vi "testarrayofclusters.vi"() -> ()   [LabVIEW 2011]
uses:
  LV JSON.lvlib
panel:
  out "Array of clusters out":T1(array[cluster])
  out "Array of clusters OK?":bool
  out "Array of clusters (JSON)":string="{\r    \"Array of clusters\": [\r        {\r            \"Numeric\": 121,\r            \"Boolean\": false,\r            \"Enum\": \"first\",\r            \"Path\": \"C:\\\\test\",\r            \"String\": \"examplestring\"\r        },\r        {\r            \"Numeric\": 121,\r            \"Boolean\": true,\r            \"Enum\": \"second\",\r            \"Path\": \"D:\\\\stest\",\r            \"String\": \"asdfasd\"\r        }\r    ]\r}"
  in  "Array of clusters":T1(array[cluster])=[{"Numeric"=121.0, "Boolean"=FALSE, "Enum"=enum."first", "Path"=path "C:/test", "String"="examplestring"}, {"Numeric"=121.0, "Boolean"=TRUE, "Enum"=enum."second", "Path"=path "D:/stest", "String"="asdfasd"}]
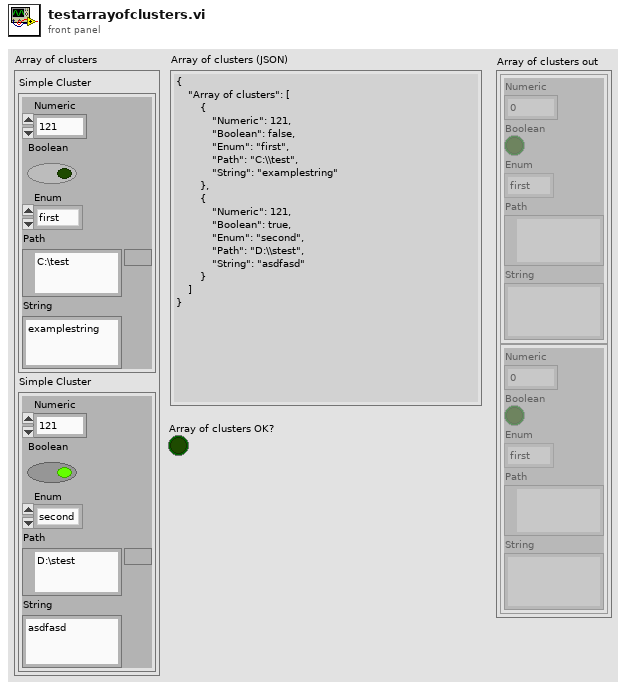
[diagram p1: front panel]
types:
  T1 = cluster{"Numeric":dbl, "Boolean":bool, "Enum":enum16{"first", "second"}, "Path":path, "String":string}[]
  T2 = cluster{"Numeric":i32, "Boolean":bool, "Enum":enum16{"first", "second"}, "Path":path, "String":string}[]
  T3 = cluster{"Numeric":bool, "Boolean":bool, "Enum":bool, "Path":bool, "String":bool}[]
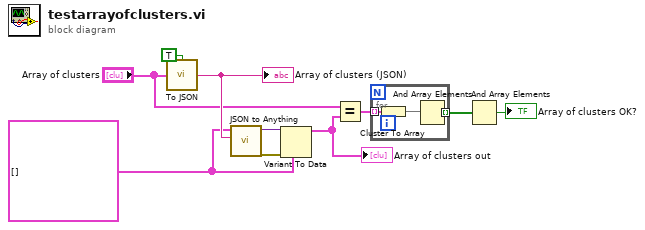
[diagram p0: block diagram]
diagram:
  w2 = T2 [] ("Array of clusters")
  n1 = call "To JSON.vi"("Anything"="Array of clusters", "Pretty Print (F)"=TRUE) -> ("JSON"=w3:string)
  "Array of clusters (JSON)" <- w3
  n2 = call "JSON to Anything.vi"("JSON Object"=w3, "Type"=w2) -> ("error out"=w6:errorcluster, "Variant"=w7:variant)  [unwired: 6 in, 2 out]
  n3 = Variant To Data(error in=w6, type=w2, Variant=w7) -> (data=w8:T2)  [unwired: 1 out]
  "Array of clusters out" <- w8
  n4 = Equal?(x="Array of clusters", y=w8) -> (x = y?=w5:T3)
  n5 = for {
    tunnel: w5 -> [w13] mode=indexing
    tunnel: [w12] -> w4 mode=indexing
    n6 = Cluster To Array(cluster=w13) -> (array=w11:bool[])
    n7 = And Array Elements(Boolean array=w11) -> (logical AND=w12:bool)
  }
  n8 = And Array Elements(Boolean array=w4) -> (logical AND=→"Array of clusters OK?":bool)
